vi "Add VIs to Class.vi"(8 "error in (no error)":errorcluster, 9 "Folder Name":string="APIs", 10 "DVR VI Paths[]":path[](array[path]), 11 "Class Path":path) -> (0 "error out":errorcluster)   [LabVIEW 2016, in "SLL Scripting.lvlib" / "SLL Class DVR API Generator.lvlib"]
uses:
  SLL Class DVR API Generator.lvlib
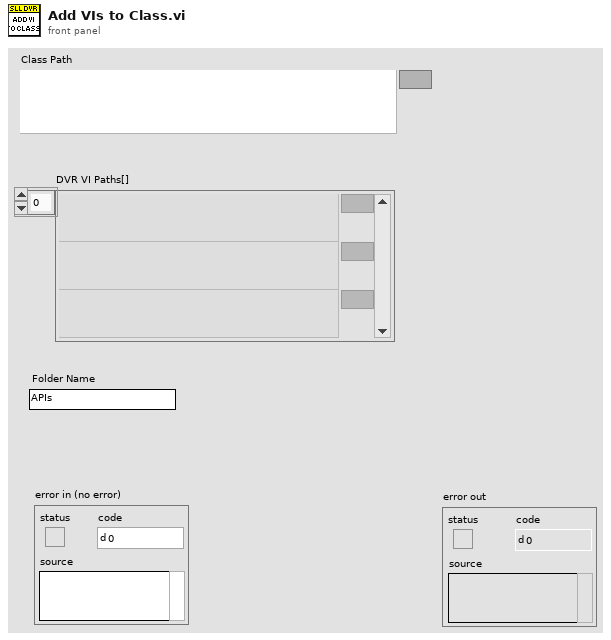
[diagram p1: front panel]
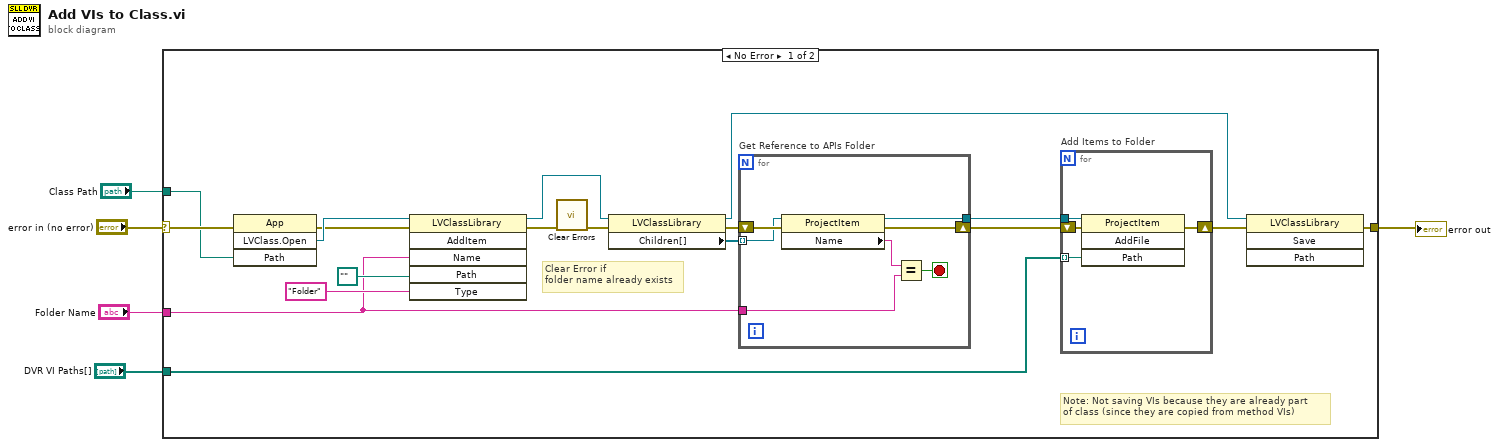
[diagram p0: block diagram]
diagram:
  n1 = case shown="No Error" "error in (no error)" {
    selector: "error in (no error)" -> [w23 w35]
    tunnel: [w8 w35] -> w4
    tunnel: "Class Path" -> [w22 _]
    tunnel: "DVR VI Paths[]" -> [w9 _]
    tunnel: "Folder Name" -> [w6 _]
    frame No Error {
      # "Note: Not saving VIs because they are already part \nof class (since they are copied from method VIs)"
      # "Clear Error if \nfolder name already exists"
      n2 = invoke class="App" method="LVClass.Open"(error in=w23, "Path"=w22) -> (error out=w17:errorcluster, "LVClass.Open"=w19:refnum<vi>)  [unwired: 2 in, 2 out]
      n3 = invoke class="LVClassLibrary" method="AddItem"(reference=w19, error in=w17, "Name"=w6, "Path"=path "", "Type"="Folder") -> (reference out=w14:refnum<vi>, error out=w21:errorcluster)  [unwired: 1 in, 4 out]
      n4 = call <vilib>:"Clear Errors.vi"("error in (no error)"=w21) -> ("error out"=w16:errorcluster)  [unwired: 5 in, 1 out]
      n5 = property class="LVClassLibrary"(reference=w14, error in=w16) -> (reference out=w7:refnum<vi>, error out=w15:errorcluster, "Children[]"=w12:refnum<vi>[])
      n6 = for "Get Reference to APIs Folder" {
        shift-right: [w33] -> w13
        shift-left: w15 -> [w34]
        tunnel: w12 -> [w32] mode=indexing
        tunnel: w6 -> [w30]
        tunnel: [w28] -> w10
        stop <- w29 stop-if-true
        n7 = property class="ProjectItem"(reference=w32, error in=w34) -> (reference out=w28:refnum<vi>, error out=w33:errorcluster, "Name"=w31:string)
        n8 = Equal?(x=w31, y=w30) -> (x = y?=w29:bool)
      }
      n9 = for "Add Items to Folder" {
        tunnel: w10 -> [w25]
        shift-right: [w26] -> w11
        shift-left: w13 -> [w27]
        tunnel: w9 -> [w24] mode=indexing
        n10 = invoke class="ProjectItem" method="AddFile"(reference=w25, error in=w27, "Path"=w24) -> (error out=w26:errorcluster)  [unwired: 1 in, 3 out]
      }
      n11 = invoke class="LVClassLibrary" method="Save"(reference=w7, error in=w11) -> (error out=w8:errorcluster)  [unwired: 2 in, 3 out]
    }
    frame Error {
    }
  }
  "error out" <- w4
